vi "ziModGetGenericHeader.vi"(8 "Error In":errorcluster, 10 "ModResults":T1, 11 "ModHandle In":T4 {"ModHandle" format="0x%08x"; "Conn" format="0x%08x"}) -> (0 "Error Out":errorcluster, 2 "ModResults":T1, 3 "ModHandle Out":T4 {"ModHandle" format="0x%08x"; "Conn" format="0x%08x"})   [LabVIEW 2018, in "Zurich Instruments LabOne.lvlib"]
doc: "Use this vi to get Double Data from a ModResult returned from ziModGetNextNode.vi. It returns an array of Double Data."
uses:
  Zurich Instruments LabOne.lvlib
  ziTypeModHandle.ctl
  ziTypeModResults.ctl
  Data/ziTypePollType.ctl
  ziTypeModGenericHeader.ctl
  ziLV32.dll
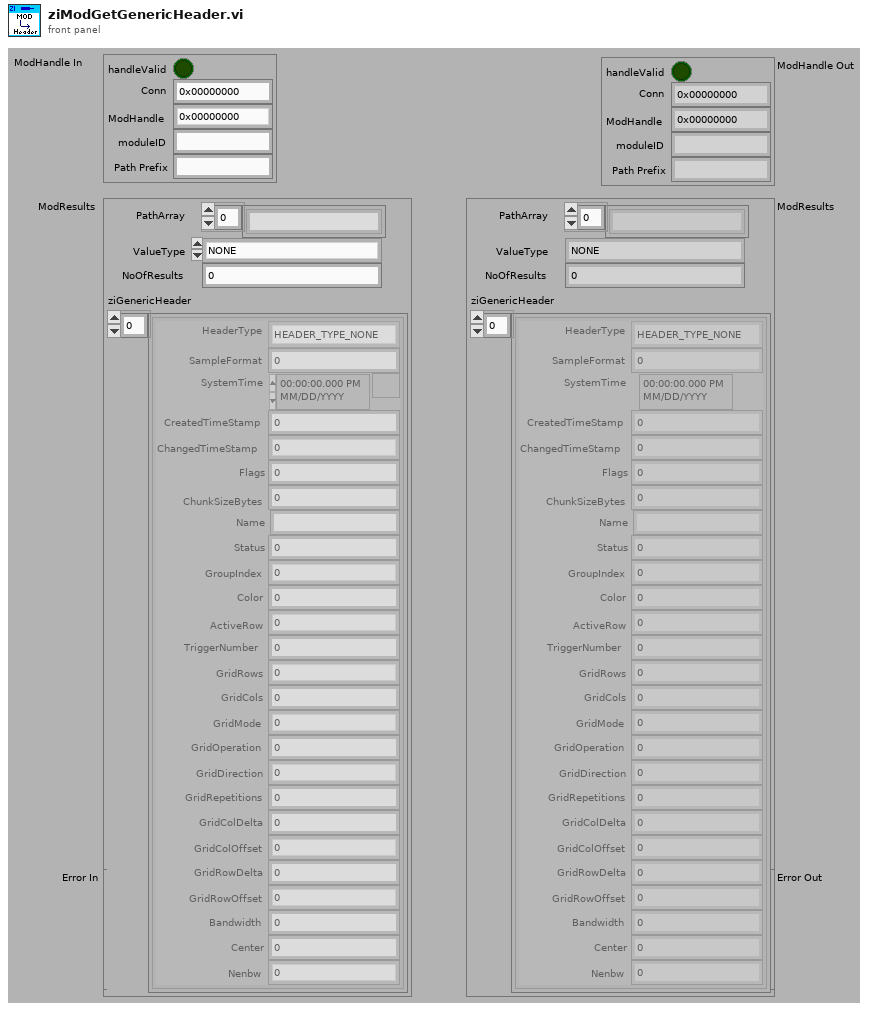
[diagram p1: front panel]
types:
  T1 = typedef "Zurich Instruments LabOne.lvlib/ziTypeModResults.ctl" = cluster{"PathArray":string[], "ValueType":T2, "NoOfResults":u64, "ziGenericHeader":T3[]}
  T2 = typedef "Zurich Instruments LabOne.lvlib/ziTypePollType.ctl" = enum16{"NONE", "DOUBLE_DATA", "INTEGER_DATA", "DEMOD_SAMPLE", "SCOPE_WAVE_HF2", "AUXIN_SAMPLE", "DIO_SAMPLE", "BYTE_ARRAY", "PWA_WAVE", "9", "10", "11", "12", "13", "14", "15", "TREE_CHANGE_DEPRI", "17", "ERROR", "19", "20", "21", "22", "23", "24", "25", "26", "27", "28", "29", "30", "31", "DOUBLE_DATA_TS", "INTEGER_DATA_TS", "34", "SCOPE_WAVE", "SCOPE_WAVE_EX", "37", "BYTE_ARRAY_TS", "39", "40", "41", "42", "43", "44", "45", "CNT_DATA", "47", "TREE_CHANGE", "49", "50", "51", "52", "53", "54", "55", "56", "57", "58", "59", "60", "61", "62", "63", "SWEEPER_DATA", "SPECTRUM_DATA", "ADVISOR_DATA", "VECTOR_DATA", "IMP_DATA"}
  T3 = typedef "Zurich Instruments LabOne.lvlib/ziTypeModGenericHeader.ctl" = cluster{"HeaderType":enum8{"HEADER_TYPE_NONE", "HEADER_TYPE_SWTRIGGER", "HEADER_TYPE_SWEEPER"}, "SampleFormat":u8, "SystemTime":timestamp, "CreatedTimeStamp":u64, "ChangedTimeStamp":u64, "Flags":u32, "ChunkSizeBytes":u64, "Name":string, "Status":u32, "GroupIndex":u32, "Color":u32, "ActiveRow":u32, "TriggerNumber":u64, "GridRows":u32, "GridCols":u32, "GridMode":u32, "GridOperation":u32, "GridDirection":u32, "GridRepetitions":u32, "GridColDelta":dbl, "GridColOffset":dbl, "GridRowDelta":dbl, "GridRowOffset":dbl, "Bandwidth":dbl, "Center":dbl, "Nenbw":dbl}
  T4 = typedef "Zurich Instruments LabOne.lvlib/ziTypeModHandle.ctl" = cluster{"handleValid":bool, "Conn":u64, "ModHandle":u64, "moduleID":string, "Path Prefix":string}
  T5 = cluster{"HeaderType":enum8{"HEADER_TYPE_NONE", "HEADER_TYPE_SWTRIGGER", "HEADER_TYPE_SWEEPER"}, "SampleFormat":u8, "SystemTime":u64, "CreatedTimeStamp":u64, "ChangedTimeStamp":u64, "Flags":u32, "ChunkSizeBytes":u64, "Name":u8[], "Status":u32, "GroupIndex":u32, "Color":u32, "ActiveRow":u32, "TriggerNumber":u64, "GridRows":u32, "GridCols":u32, "GridMode":u32, "GridOperation":u32, "GridDirection":u32, "GridRepetitions":u32, "GridColDelta":dbl, "GridColOffset":dbl, "GridRowDelta":dbl, "GridRowOffset":dbl, "Bandwidth":dbl, "Center":dbl, "Nenbw":dbl}
  T6 = enum8{"HEADER_TYPE_NONE", "HEADER_TYPE_SWTRIGGER", "HEADER_TYPE_SWEEPER"}
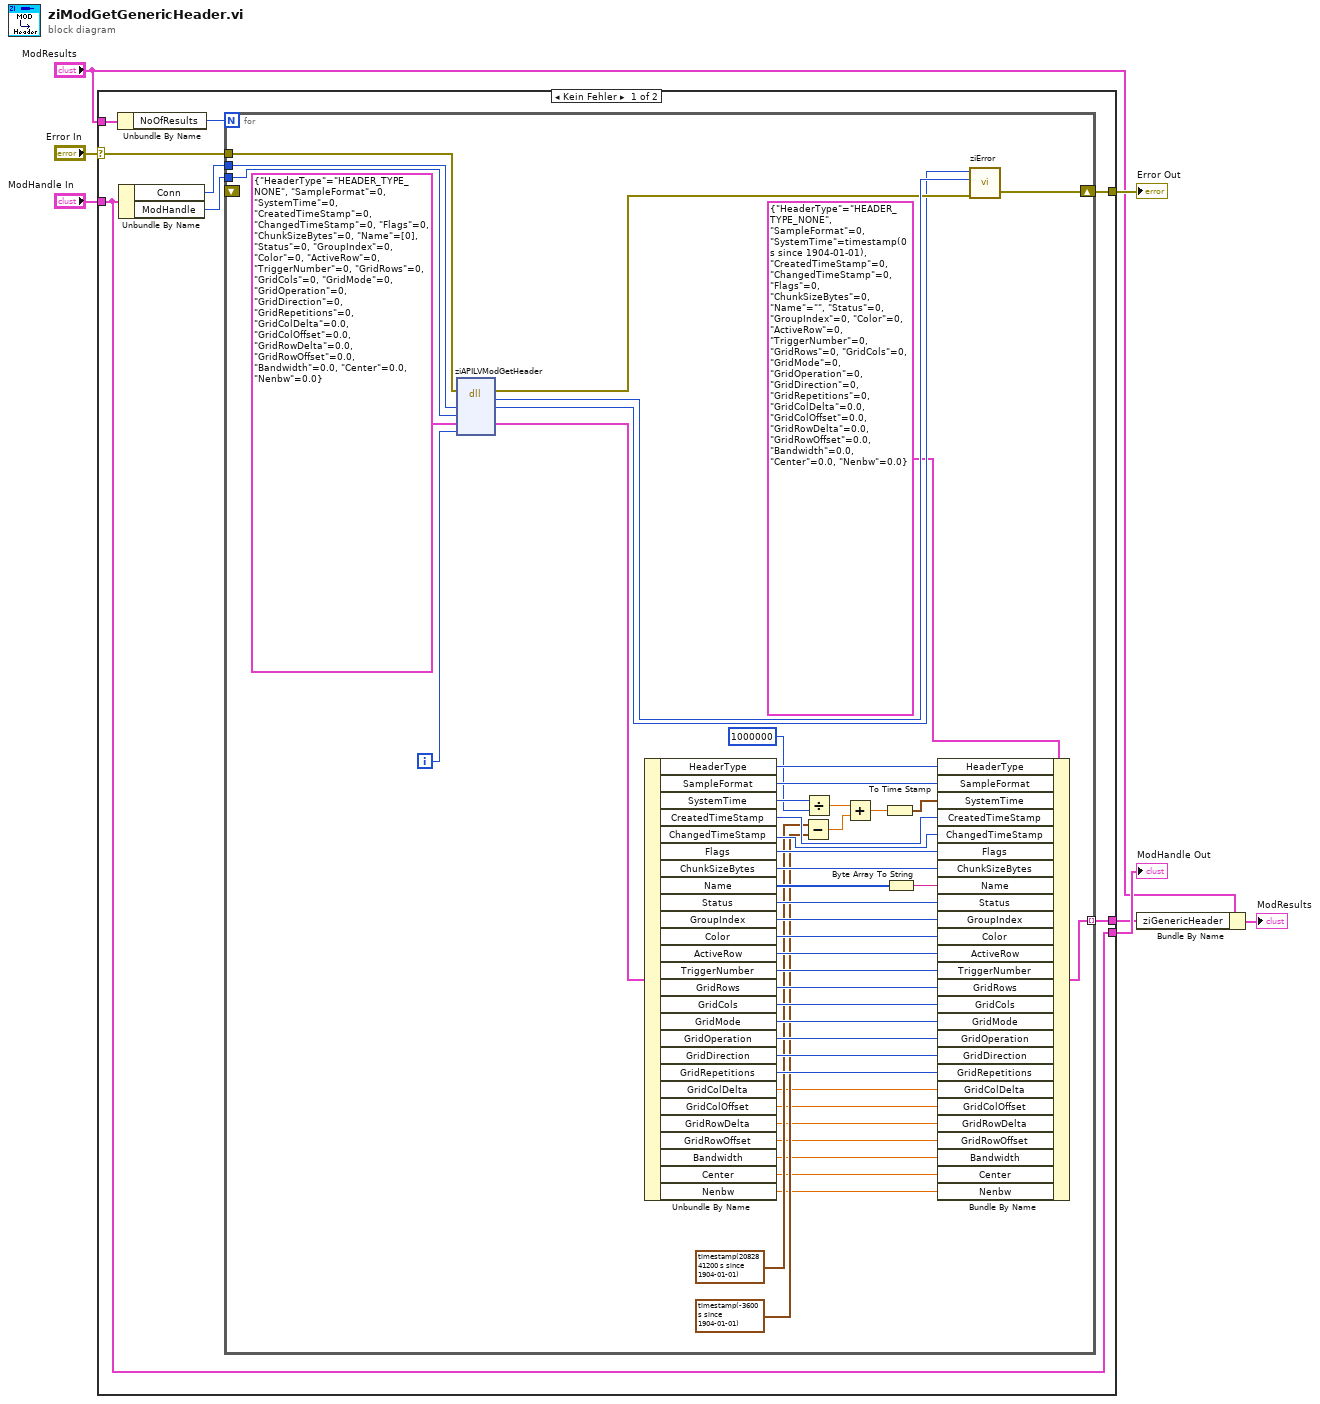
[diagram p0: block diagram]
diagram:
  n1 = case shown="Kein Fehler" "Error In" {
    selector: "Error In" -> [w11 w62]
    tunnel: [w12 w62] -> w4
    tunnel: [w10 w63] -> w6
    tunnel: "ModHandle In" -> [w10 w63]
    tunnel: "ModResults" -> [w13 _]
    tunnel: [w9 _] -> w1
    frame No Error {
      n2 = Unbundle By Name(w13) -> ("NoOfResults"=w8:u64)
      n3 = Unbundle By Name(w10) -> ("Conn"=w15:u64, "ModHandle"=w14:u64)
      n4 = for {
        N: w8 -> [_]
        tunnel: w15 -> [w61]
        tunnel: w14 -> [w60]
        tunnel: w11 -> [w58]
        tunnel: [w52] -> w9 mode=indexing
        shift-right: [w59] -> w12
        shift-left: _ -> [_]
        i -> [w55]
        n5 = dll-call lib="ziLV*.*" fn="ziAPILVModGetHeader" label="ziAPILVModGetGenericHeader"(error in=w58, "Conn"=w61, "ModHandle"=w60, T5 {"HeaderType"=enum."HEADER_TYPE_NONE", "SampleFormat"=0, "SystemTime"=0, "CreatedTimeStamp"=0, "ChangedTimeStamp"=0, "Flags"=0, "ChunkSizeBytes"=0, "Name"=[0], "Status"=0, "GroupIndex"=0, "Color"=0, "ActiveRow"=0, "TriggerNumber"=0, "GridRows"=0, "GridCols"=0, "GridMode"=0, "GridOperation"=0, "GridDirection"=0, "GridRepetitions"=0, "GridColDelta"=0.0, "GridColOffset"=0.0, "GridRowDelta"=0.0, "GridRowOffset"=0.0, "Bandwidth"=0.0, "Center"=0.0, "Nenbw"=0.0} ("ziModResults"), "chunk_idx"=w55) -> (error out=w56:errorcluster, "return type"=w57:u32, "Conn"=w54:u64, w51:T5)  [unwired: 4 in, 1 out]
        n6 = Unbundle By Name(w51) -> ("HeaderType"=w47:T6, "SampleFormat"=w46:u8, "SystemTime"=w30:u64, "CreatedTimeStamp"=w45:u64, "ChangedTimeStamp"=w44:u64, "Flags"=w43:u32, "ChunkSizeBytes"=w42:u64, "Name"=w49:u8[], "Status"=w41:u32, "GroupIndex"=w40:u32, "Color"=w39:u32, "ActiveRow"=w38:u32, "TriggerNumber"=w37:u64, "GridRows"=w36:u32, "GridCols"=w35:u32, "GridMode"=w34:u32, "GridOperation"=w33:u32, "GridDirection"=w32:u32, "GridRepetitions"=w31:u32, "GridColDelta"=w16:dbl, "GridColOffset"=w17:dbl, "GridRowDelta"=w18:dbl, "GridRowOffset"=w19:dbl, "Bandwidth"=w20:dbl, "Center"=w21:dbl, "Nenbw"=w22:dbl)
        n7 = Subtract(x=timestamp(2082841200 s since 1904-01-01), y=timestamp(-3600 s since 1904-01-01)) -> (x-y=w27:dbl)
        n8 = Divide(x=w30, y=u64 1000000) -> (x/y=w26:dbl)
        n9 = Add(x=w26, y=w27) -> (x+y=w25:dbl)
        n10 = To Time Stamp(1:w25) -> (0:w24:timestamp)
        n11 = Byte Array To String(unsigned byte array=w49) -> (string=w50:string)
        n12 = Bundle By Name(cluster=T3 {"HeaderType"=enum."HEADER_TYPE_NONE", "SampleFormat"=0, "SystemTime"=timestamp(0 s since 1904-01-01), "CreatedTimeStamp"=0, "ChangedTimeStamp"=0, "Flags"=0, "ChunkSizeBytes"=0, "Name"="", "Status"=0, "GroupIndex"=0, "Color"=0, "ActiveRow"=0, "TriggerNumber"=0, "GridRows"=0, "GridCols"=0, "GridMode"=0, "GridOperation"=0, "GridDirection"=0, "GridRepetitions"=0, "GridColDelta"=0.0, "GridColOffset"=0.0, "GridRowDelta"=0.0, "GridRowOffset"=0.0, "Bandwidth"=0.0, "Center"=0.0, "Nenbw"=0.0} ("ziModResults"), "HeaderType"=w47, "SampleFormat"=w46, "SystemTime"=w24, "CreatedTimeStamp"=w45, "ChangedTimeStamp"=w44, "Flags"=w43, "ChunkSizeBytes"=w42, "Name"=w50, "Status"=w41, "GroupIndex"=w40, "Color"=w39, "ActiveRow"=w38, "TriggerNumber"=w37, "GridRows"=w36, "GridCols"=w35, "GridMode"=w34, "GridOperation"=w33, "GridDirection"=w32, "GridRepetitions"=w31, "GridColDelta"=w16, "GridColOffset"=w17, "GridRowDelta"=w18, "GridRowOffset"=w19, "Bandwidth"=w20, "Center"=w21, "Nenbw"=w22) -> (w52:T3)
        n13 = call "ziError.vi"("Conn"=w54, "ziErrorCode"=w57, "Error In"=w56) -> ("Error Out"=w59:errorcluster)  [unwired: 2 in, 1 out]
      }
    }
    frame Error {
    }
  }
  "Error Out" <- w4
  "ModHandle Out" <- w6
  n14 = Bundle By Name(cluster="ModResults", "ziGenericHeader"=w1) -> (→"ModResults":T1)
